vi "EventDispose.vi"(8 "error in (no error)":errorcluster, 11 "Execute":refnum<class "Execute.lvclass">) -> (0 "error out":errorcluster, 3 "Execute":refnum<class "Execute.lvclass">)   [LabVIEW 2018, in "QMH_Class.lvlib" / "TestManager.lvlib" / "Execute.lvclass"]
uses:
  Execute.lvclass
  Execute.lvclass/Execute.ctl
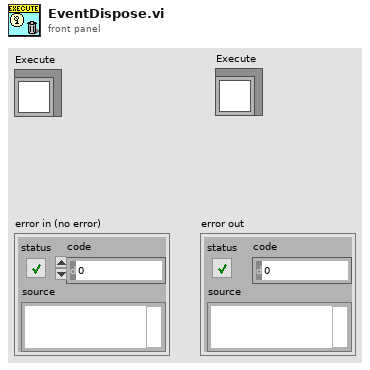
[diagram p1: front panel]
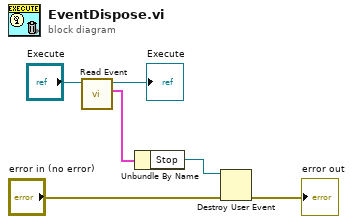
[diagram p0: block diagram]
diagram:
  n1 = call "Read Event.vi"("Execute"="Execute") -> ("Event"=w4:cluster{"Stop":refnum<user-event>}, "Execute"=→"Execute":refnum<class "Execute.lvclass">)  [unwired: 8 in, 1 out]
  n2 = Unbundle By Name(w4) -> ("Stop"=w3:refnum<user-event>)
  n3 = Destroy User Event(user event=w3, error in="error in (no error)") -> (error out=→"error out":errorcluster)
